vi "Read Close Button Image.vi"(8 "error in (no error)":errorcluster, 11 "QMenu Class in":refnum<class "QMenu Class.lvclass">) -> (0 "error out":errorcluster, 2 "Close Button Image":T1, 3 "QMenu Class out":refnum<class "QMenu Class.lvclass">)   [LabVIEW 2020, in "QTab.lvlib" / "QMenu Class.lvclass"]
uses:
  QMenu Class.lvclass
  <vilib>/picture/picture.llb/imagedata.ctl
  QMenu Class.lvclass/QMenu Class.ctl
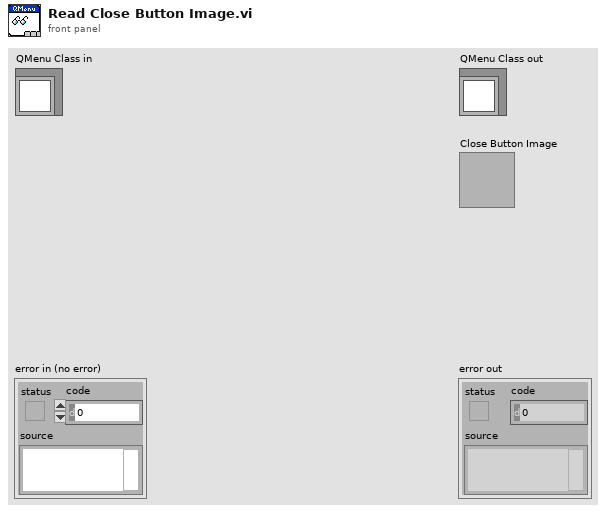
[diagram p1: front panel]
types:
  T1 = typedef "imagedata.ctl" = cluster{"image type":i32, "image depth":i32, "image":u8[], "mask":u8[], "colors":u32[], "Rectangle":cluster{"left":i16, "top":i16, "right":i16, "bottom":i16}}
  T2 = typedef "QTab.lvlib/QMenu Class.lvclass/Image Data.ctl" = cluster{"Button Image":T1, "Close Button Image":T1, "Left Button Image":T1, "Right Button Image":T1}
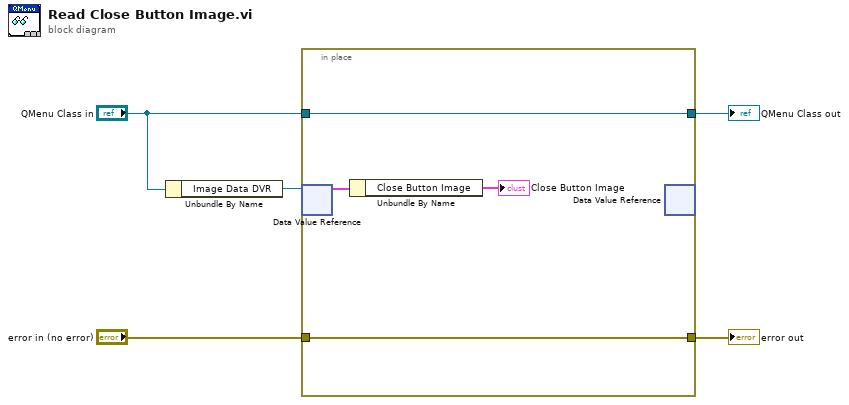
[diagram p0: block diagram]
diagram:
  n1 = Unbundle By Name("QMenu Class in") -> ("Image Data DVR"=w4:refnum<data-value>)
  n2 = in-place {
    in-place-border: "QMenu Class in" -> [w9]
    in-place-border: "error in (no error)" -> [w8]
    in-place-border: [w9] -> w2
    in-place-border: [w8] -> w1
    n3 = in-place-dvr #1(w4) -> (w7:T2)  [unwired: 1 out]
    n4 = Unbundle By Name(w7) -> ("Close Button Image"=→"Close Button Image":T1)
    n5 = in-place-dvr #1() -> ()  [unwired: 1 in, 2 out]
  }
  "error out" <- w1
  "QMenu Class out" <- w2
